vi "Pre Launch Init.vi"(11 "Nested in":refnum<class "Items.lvclass">) -> (0 "error out":errorcluster, 3 "Nested out":refnum<class "Items.lvclass">)   [LabVIEW 2020, in "Items.lvlib" / "Items.lvclass"]
doc: "(<B>Filename</B>: Actor Framework.lvlib:Actor.lvclass:Pre Launch Init.vi)\n\nDefines behavior that occurs after the Launch Nested Actor method is invoked but before the actor's Actor Core method begins running.\n\nBy default, this method does nothing. A descendant class may override it to define behavior."
uses:
  Items.lvclass
  C:/Program Files (x86)/National Instruments/LabVIEW 2020/vi.lib/ActorFramework/Actor/Actor.lvclass
  Items.lvclass/Items.ctl
  <vilib>/ActorFramework/Actor/Actor.lvclass/Actor.ctl
  <vilib>/ActorFramework/Message Enqueuer/Message Enqueuer.lvclass/Message Enqueuer.ctl
  <vilib>/ActorFramework/Message Enqueuer/Init from Existing Queue.vi
  <vilib>/ActorFramework/Message Enqueuer/Enqueue.vi
  Items Messages/Draw Actor Core UI on SubPanel Msg/Draw Actor Core UI on SubPanel Msg.lvclass
  C:/Program Files (x86)/National Instruments/LabVIEW 2020/vi.lib/ActorFramework/Message/Message.lvclass
  <vilib>/ActorFramework/Message Priority Queue/Priority Enqueue.vi
  <vilib>/ActorFramework/Message Enqueuer/Message Enqueuer.lvclass
  <vilib>/ActorFramework/Actor/Actor.lvclass
  Items Messages/Load Inventory Msg/Load Inventory Msg.lvclass
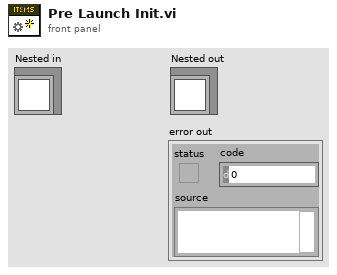
[diagram p1: front panel]
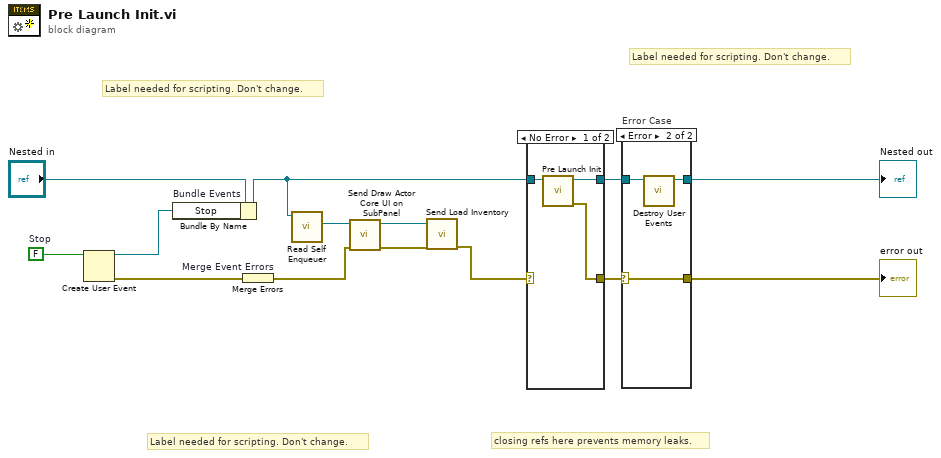
[diagram p0: block diagram]
diagram:
  w13 = FALSE  # Stop
  # "Label needed for scripting. Don't change."
  # "Label needed for scripting. Don't change."
  # "Label needed for scripting. Don't change."
  # "closing refs here prevents memory leaks."
  n1 = Create User Event(user event datatype=w13) -> (user event=w10:refnum<user-event>, error out=w12:errorcluster)  [unwired: 1 in]
  n2 = Bundle By Name "Bundle Events"(cluster="Nested in", "Stop"=w10) -> (w6:refnum<class "Items.lvclass">)
  n3 = Merge Errors "Merge Event Errors"(w12) -> (w4:errorcluster)
  n4 = call <vilib>:"Read Self Enqueuer.vi"("Actor"=w6) -> ("Self Enqueuer"=w5:refnum<class "Message Enqueuer.lvclass">)  [unwired: 10 in]
  n5 = call "Send Draw Actor Core UI on SubPanel.vi"("error in (no error)"=w4, "Message Enqueuer"=w5) -> ("error out"=w2:errorcluster, "Message Enqueuer out"=w3:refnum<class "Message Enqueuer.lvclass">)  [unwired: 8 in]
  n6 = call "Send Load Inventory.vi"("error in (no error)"=w2, "Message Enqueuer"=w3) -> ("error out"=w1:errorcluster)  [unwired: 8 in, 1 out]
  n7 = case shown="No Error" w1 {
    selector: w1 -> [_ w19]
    tunnel: [w17 w18] -> w8
    tunnel: w6 -> [w16 w18]
    tunnel: [w15 w19] -> w7
    frame No Error {
      n8 = call-parent "Pre Launch Init.vi"("Actor in"=w16) -> ("error out"=w15:errorcluster, "Actor out"=w17:refnum<class "Items.lvclass">)  [unwired: 9 in]
    }
    frame Error {
    }
  }
  n9 = case "Error Case" shown="Error" w7 {
    selector: w7 -> [w20 w24]
    tunnel: w8 -> [w21 w23]
    tunnel: [w21 w22] -> w11
    tunnel: [w20 w24] -> w9
    frame No Error {
    }
    frame Error {
      n10 = call "Destroy User Events.vi"("UI Template in"=w23) -> ("UI Template out"=w22:refnum<class "Items.lvclass">)  [unwired: 10 in]
    }
  }
  "error out" <- w9
  "Nested out" <- w11
